vi "mW_EIOTemp_check.vi"(10 "Temp Gradients":refnum<vi>, 11 "EIO temp":refnum<vi>) -> (3 "Temp alarms":bool)   [LabVIEW 2019]
panel:
  in  "y":dbl=-0.1
  out "Temp Gradients":dbl[](array[numeric])
  in  "temp":dbl=33.0
  out "EIO top plate":dbl
  out "First wave guid":dbl
  out "Splitter Temp":dbl
  out "T_array":dbl[](array[numeric])
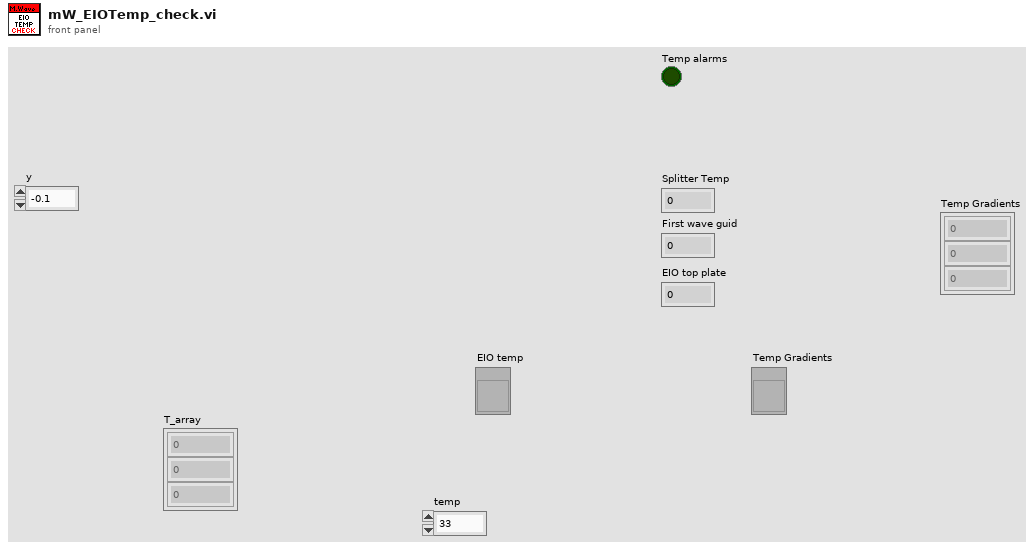
[diagram p1: front panel]
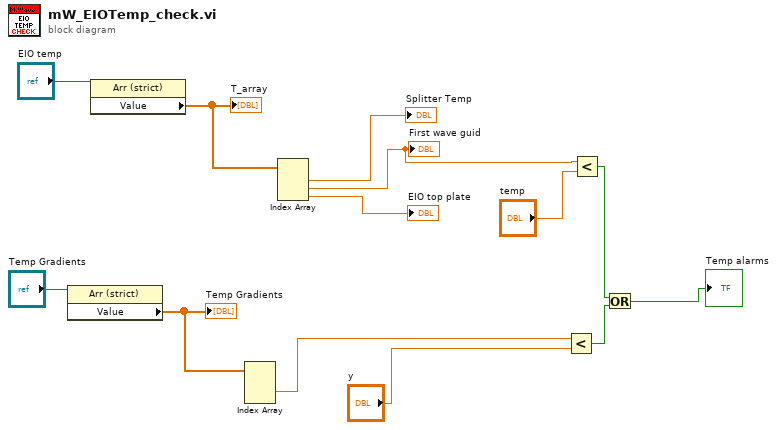
[diagram p0: block diagram]
diagram:
  n1 = property class="Arr (strict)"(reference="Temp Gradients") -> ("Value"=w6:dbl[])  [unwired: 1 in, 2 out]
  "Temp Gradients" <- w6
  n2 = property class="Arr (strict)"(reference="EIO temp") -> ("Value"=w12:dbl[])  [unwired: 1 in, 2 out]
  "T_array" <- w12
  n3 = Index Array(array=w6) -> (element #2=w5:dbl)  [unwired: 3 in, 2 out]
  n4 = Index Array(array=w12) -> (element #1=→"Splitter Temp":dbl, element #2=w9:dbl, element #3=→"EIO top plate":dbl)  [unwired: 3 in]
  "First wave guid" <- w9
  n5 = Less?(x=w5, y="y") -> (x < y?=w3:bool)
  n6 = Less?(x=w9, y="temp") -> (x < y?=w2:bool)
  n7 = Or(x=w2, y=w3) -> (x .or. y?=→"Temp alarms":bool)
